vi "Yokogawa GX20 Start Compute Example RS422.vi"() -> ()   [LabVIEW 2020]
doc: "This example shows how to start compute."
uses:
  <instrlib>/Yokogawa GX Series/Yokogawa GX Series.lvlib
panel:
  in  "User ID (\"\")":string
  in  "Password (\"\")":string
  in  "User Name (\"\")":string
  in  "Serial Configuration":T1={"Baud Rate"=9600, "Parity"=2, "Data Bits"=8, "Flow Control"=0} {"Flow Control" items=["None", "XON/XOFF", "RTS/CTS", "XON/XOFF & RTS/CTS"]; "Data Bits" items=["7"=7, "8"=8]; "Parity" items=["None", "Odd", "Even"]; "Baud Rate" items=["1200"=1200, "2400"=2400, "4800"=4800, "9600"=9600, "19200"=19200, "38400"=38400, "57600"=57600, "115200"=115200]}
  in  "VISA resource name":refnum<visa-resource-name>
  # "(c) 2013-2018 Yokogawa Electric Corporation.  ALL RIGHTS RESERVED."
  # "GX10/GX20/GP10/GP20/GM10 PAPERLESS RECORDER"
  # "When you run this VI, GX/GP/GM starts compute."
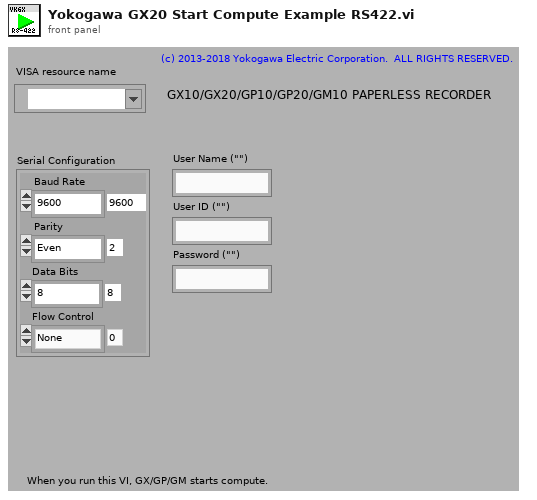
[diagram p1: front panel]
types:
  T1 = cluster{"Baud Rate":u32, "Parity":u16, "Data Bits":u16, "Flow Control":u16}
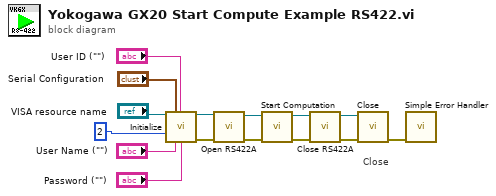
[diagram p0: block diagram]
diagram:
  # "Close"
  n1 = call <instrlib>:"Initialize.vi"("VISA resource name IN"="VISA resource name", "Serial Configuration"="Serial Configuration", "User ID (\"\")"="User ID (\"\")", "Serial Auth Type (0: Not Auth)"=2, "User Name (\"admin\")"="User Name (\"\")", "Password (\"\")"="Password (\"\")") -> ("VISA resource name out"=w12:refnum<visa-resource-name>, "error out"=w13:errorcluster)  [unwired: 8 in]
  n2 = call <instrlib>:"Open RS422A.vi"("error in (no error)"=w13, "VISA resource name"=w12) -> ("error out"=w6:errorcluster, "VISA resource name out"=w11:refnum<visa-resource-name>)  [unwired: 8 in]
  n3 = call <instrlib>:"Start Computation.vi"("error in (no error)"=w6, "VISA resource name"=w11) -> ("error out"=w9:errorcluster, "VISA resource name out"=w8:refnum<visa-resource-name>)  [unwired: 8 in]
  n4 = call <instrlib>:"Close RS422A.vi"("error in (no error)"=w9, "VISA resource name"=w8) -> ("error out"=w10:errorcluster, "VISA resource name out"=w7:refnum<visa-resource-name>)  [unwired: 8 in]
  n5 = call <instrlib>:"Close.vi"("error in (no error)"=w10, "VISA resource name"=w7) -> ("error out"=w15:errorcluster)  [unwired: 9 out]
  n6 = call <vilib>:"Simple Error Handler.vi"("error in (no error)"=w15) -> ()  [unwired: 1 in, 8 out]
